vi "gantry_rot_stop.vi"(8 "Rapid stop?":bool, 11 "VISA resource name":refnum<visa-resource-name>) -> (3 "VISA resource name out":refnum<visa-resource-name>)   [LabVIEW 2021]
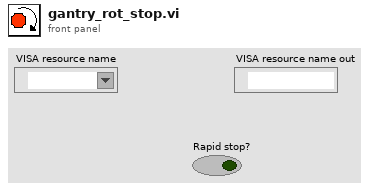
[diagram p1: front panel]
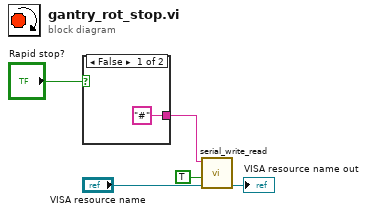
[diagram p0: block diagram]
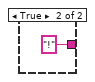
[diagram p2: hidden frame]
diagram:
  n1 = case shown="False" "Rapid stop?" {
    tunnel: ["#" ("write buffer") "!" ("write buffer")] -> w4
    frame False {
    }
    frame True {
    }
  }
  n2 = call "serial_write_read.vi"("VISA resource name"="VISA resource name", "Clear buffer"=TRUE, "write buffer"=w4) -> ("VISA resource name out"=→"VISA resource name out":refnum<visa-resource-name>)  [unwired: 7 in, 1 out]
